vi "Build core.vi"(6 "Previous Build's Artifacts":refnum<class "Build Artifact.lvclass">[](array[class]), 7 "Progress":refnum<class "Progress.lvclass">, 8 "error in (no error)":errorcluster, 10 "Build Cache":refnum<class "Build Cache.lvclass">, 11 "Build Item in":refnum<class "Create ZIP Step.lvclass">) -> (0 "error out":errorcluster, 1 "Explore Path":path, 2 "Build Results":T1, 4 "New Artifacts":refnum<class "Build Artifact.lvclass">[](array[class]))   [LabVIEW 2019, in "ZIP.lvlib" / "Create ZIP Step.lvclass"]
doc: "Performs all the necessary build actions for the build step.\n\nCopyright: MGI 2016\nAuthor: Derek Trepanier"
uses:
  Create ZIP Step.lvclass
  libs/Solution.lvlibp/Solution/Progress/Progress.lvclass
  libs/Solution.lvlibp/Solution/Build Artifact/Build Artifact.lvclass
  libs/Solution.lvlibp/Solution/Build Item/Build Result.ctl
  libs/Solution.lvlibp/Solution/Build Cache/Build Cache.lvclass
  Create ZIP Step.lvclass/Create ZIP Step.ctl
  libs/Solution.lvlibp/Solution/Build Item/Build Step.lvclass
  libs/Project.lvlibp/Project/Binary File/Binary File.lvclass
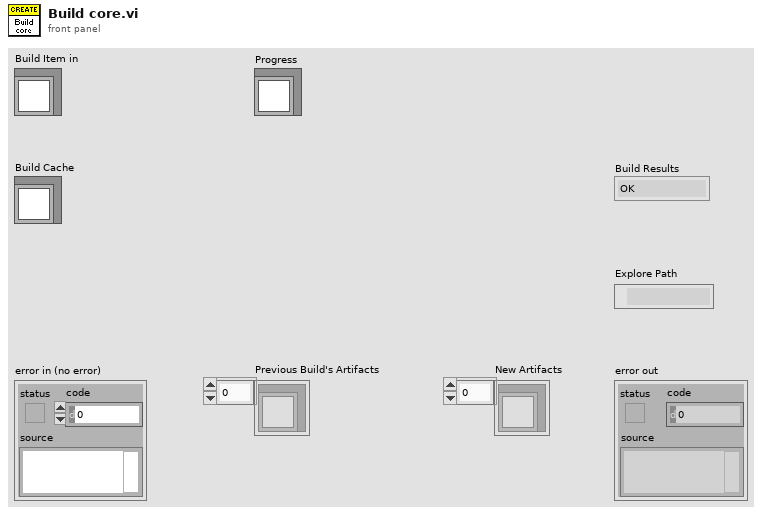
[diagram p1: front panel]
types:
  T1 = typedef "Solution.lvlibp/Build Step.lvclass/Build Result.ctl" = enum16{"OK", "Skipped", "Error"}
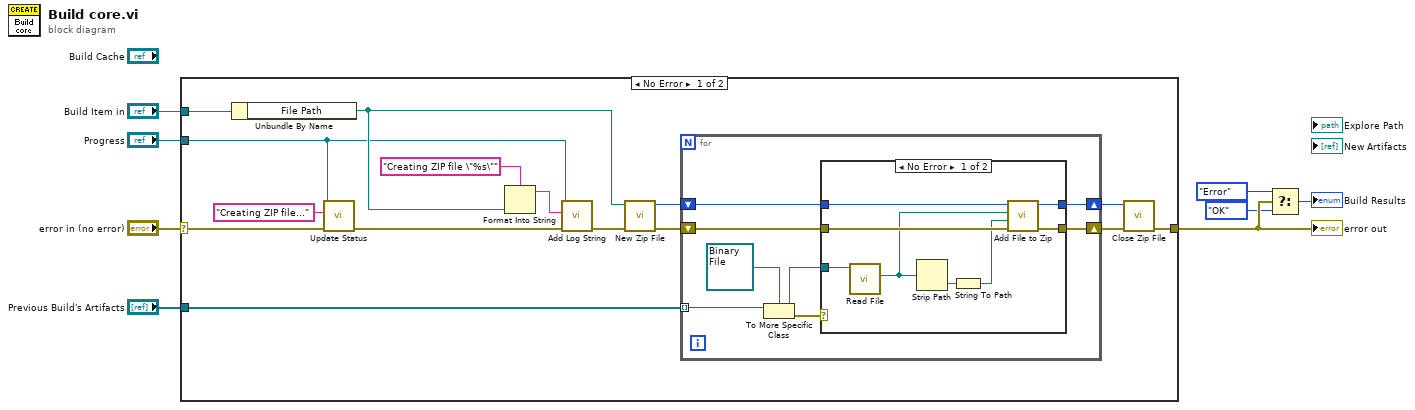
[diagram p0: block diagram]
diagram:
  n1 = case shown="No Error" "error in (no error)" {
    selector: "error in (no error)" -> [w16 w42]
    tunnel: "Build Item in" -> [w23 _]
    tunnel: [w21 w42] -> w6
    tunnel: "Progress" -> [w14 _]
    tunnel: "Previous Build's Artifacts" -> [w9 _]
    frame No Error {
      n2 = Unbundle By Name(w23) -> ("File Path"=w17:path)
      n3 = call "Update Status.vi"("error in (no error)"=w16, "Status String"="Creating ZIP file...", "Progress in"=w14) -> ("error out"=w15:errorcluster)  [unwired: 8 in]
      n4 = Format Into String(format string="Creating ZIP file \"%s\"", w17) -> (resulting string=w18:string)  [unwired: 2 in, 1 out]
      n5 = call "Add Log String.vi"("error in (no error)"=w15, "Log Item"=w18, "Progress in"=w14) -> ("error out"=w20:errorcluster)  [unwired: 8 in]
      n6 = call <vilib>:"New Zip File.vi"("error in (no error)"=w20, "target"=w17) -> ("error out"=w22:errorcluster, "zip file out"=w11:i64)  [unwired: 3 in, 1 out]
      n7 = for {
        shift-right: [w30] -> w12
        shift-left: w22 -> [w31]
        shift-right: [w28] -> w10
        shift-left: w11 -> [w29]
        tunnel: w9 -> [w27] mode=indexing
        n8 = To More Specific Class(target class=refnum<class "Binary File.lvclass"> refnum ("Project.lvlibp:Binary File.lvclass"), reference=w27) -> (specific class reference=w24:refnum<class "Binary File.lvclass">, error out=w25:errorcluster)  [unwired: 1 in]
        n9 = case shown="No Error" w25 {
          tunnel: w31 -> [w39 w40]
          tunnel: [w38 w40] -> w30
          tunnel: w29 -> [w37 w41]
          tunnel: [w36 w41] -> w28
          tunnel: w24 -> [w35 _]
          frame No Error {
            n10 = call "Read File.vi"("Binary File in"=w35) -> ("File"=w34:path)  [unwired: 8 in, 2 out]
            n11 = Strip Path(path=w34) -> (name=w33:string)  [unwired: 1 out]
            n12 = String To Path(string=w33) -> (path=w32:path)
            n13 = call <vilib>:"Add File to Zip.vi"("error in (no error)"=w39, "destination path in zip"=w32, "source file path"=w34, "zip file in"=w37) -> ("error out"=w38:errorcluster, "zip file out"=w36:i64)  [unwired: 6 in]
          }
          frame Error {
          }
        }
      }
      n14 = call <vilib>:"Close Zip File.vi"("error in (no error)"=w12, "zip file in"=w10) -> ("error out"=w21:errorcluster)  [unwired: 5 in]
    }
    frame Error {
    }
  }
  "error out" <- w6
  n15 = Select(t=Build_Result."Error" ("Build Results"), s=w6, f=Build_Result."OK") -> (s? t:f=→"Build Results":T1)
